vi "SendBufferIn.vi"(1 "remote":bool, 2 "ID":u32 format="%04x", 4 "ExtFrame":bool, 5 "数据":u8[](array[numeric])) -> ()   [LabVIEW 2011]
uses:
  _USB_CAN_SEND_BUFF_UNIT_.ctl
  _USB_CAN_GLOBAL_.vi
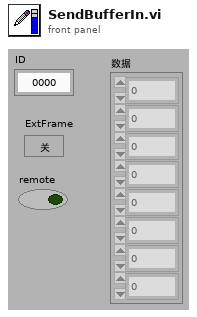
[diagram p1: front panel]
types:
  T1 = typedef "_USB_CAN_SEND_BUFF_UNIT_.ctl" = cluster{"datalen":u8, "data":u8[], "id":u8[], "extended":bool, "remote":bool}
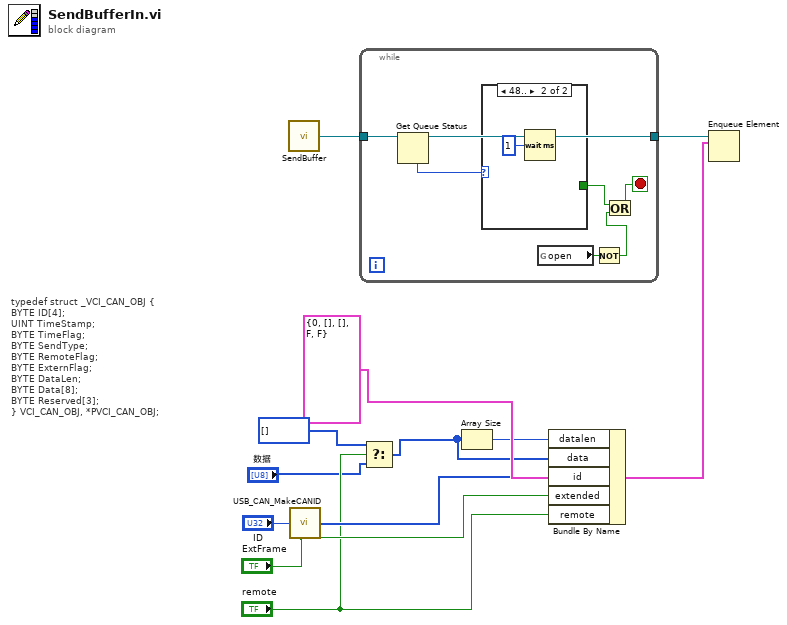
[diagram p0: block diagram]
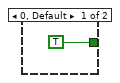
[diagram p2: hidden frame]
diagram:
  # "typedef struct _VCI_CAN_OBJ { \nBYTE ID[4];\nUINT TimeStamp; \nBYTE TimeFlag;\nBYTE SendType; \nBYTE RemoteFlag; \nBYTE ExternFlag; \nBYTE DataLen; \nBYTE Data[8]; \nBYTE Reserved[3];\n} VCI_CAN_OBJ, *PVCI_CAN_OBJ;"
  n1 = call "SendBuffer.vi"() -> ("VCI_CAN_BUF_T"=w7:refnum<queue>)  [unwired: 1 in]
  n2 = call "USB_CAN_MakeCANID.vi"("ID"="ID", "ExtFrame"="ExtFrame") -> ("IDS"=w10:u8[])  [unwired: 3 in]
  n3 = while {
    tunnel: w7 -> [w19]
    tunnel: [w18] -> w6
    stop <- w15 stop-if-true
    n4 = Get Queue Status(queue=w19) -> (queue out=w18:refnum<queue>, # elements in queue=w17:i32)  [unwired: 2 in, 6 out]
    n5 = case shown="48.." w17 {
      tunnel: [TRUE _] -> w16
      frame 0, Default {
      }
      frame 48.. {
        n6 = Wait (ms)(milliseconds to wait=u32 1 ("等待时间（毫秒）")) -> ()  [unwired: 1 out]
      }
    }
    n7 = global read "_USB_CAN_GLOBAL_.vi" "open"() -> (w14:bool)
    n8 = Not(x=w14) -> (.not. x?=w13:bool)
    n9 = Or(x=w16, y=w13) -> (x .or. y?=w15:bool)
  }
  n10 = Select(t=u8[] [], s="remote", f="数据") -> (s? t:f=w1:u8[])
  n11 = Array Size(array=w1) -> (size(s)=w8:i32)
  n12 = Bundle By Name(cluster=T1 {"datalen"=0, "data"=[], "id"=[], "extended"=FALSE, "remote"=FALSE} ("VCI_CAN_BUF_T"), "datalen"=w8, "data"=w1, "id"=w10, "extended"="ExtFrame", "remote"="remote") -> (w5:T1)
  n13 = Enqueue Element(queue=w6, element=w5) -> ()  [unwired: 2 in, 3 out]
